vi "2100_Bridge_Read RFFE_w_Waveform_Publish Data.vi"(0 "Semiconductor Module Context":T2, 1 "Pins":string[](array[string])=["CLK", "SDA"], 2 "USID":T1=8 max=15, 3 "Reg Address":u8=6 format="%.0x", 5 "Error In":errorcluster, 6 "Read_Mode":enum16{"Reg_Read", "Bit_Read"}(ring), 7 "Bit_Location(LSB)":u8=7 max=7, 8 "Publish_Data?":bool, 9 "#ofBits":u8=1 min=1 max=8, 10 "Published Data Id":string) -> (14 "Converted Data":T3 {"Register" max=31 format="%.0x"; "Slave Address" max=15 format="%.0x"}, 15 "Reg Value":u8 format="%.0b", 19 "Error Out":errorcluster)   [LabVIEW 2013]
uses:
  <vilib>/NI_TestStand_SemiconductorModule/NI_TestStand_Semiconductor_Module.lvlibp/PinMap/General/SemiconductorModuleContext.ctl
  Controls/USID.ctl
  Controls/Reg_Address_Data.ctl
  <vilib>/NI_TestStand_SemiconductorModule/NI_TestStand_Semiconductor_Module.lvlibp/PinMap/General/Publish/PublishDataDoubleFunctionalTest.vi
  <vilib>/NI_TestStand_SemiconductorModule/NI_TestStand_Semiconductor_Module.lvlibp
panel:
  # "Specific Bit Readback"
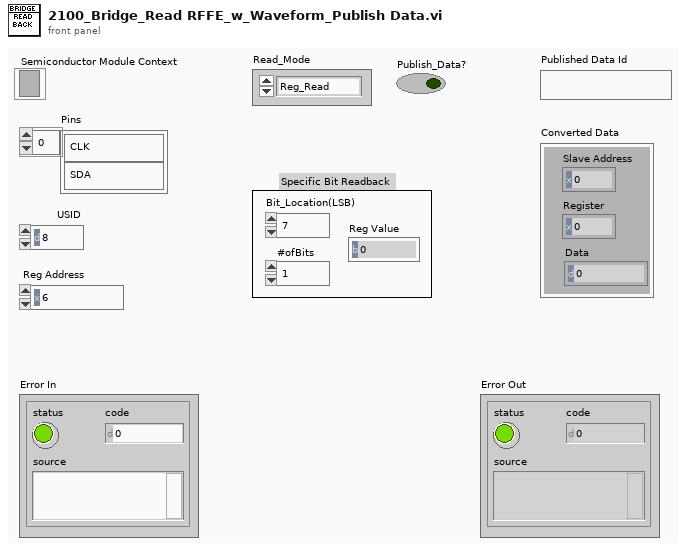
[diagram p1: front panel]
types:
  T1 = typedef "USID.ctl" = u8
  T2 = typedef "NI_TestStand_Semiconductor_Module.lvlibp/SemiconductorModuleContext.ctl" = refnum<k7>
  T3 = cluster{"Slave Address":u8, "Register":u8, "Data":u8}
  T4 = typedef "Reg_Address_Data.ctl" = cluster{"Address":u8, "Data":u8}
  T5 = cluster{"First Reg Address":u8, "Num of Reg to Read":u8}
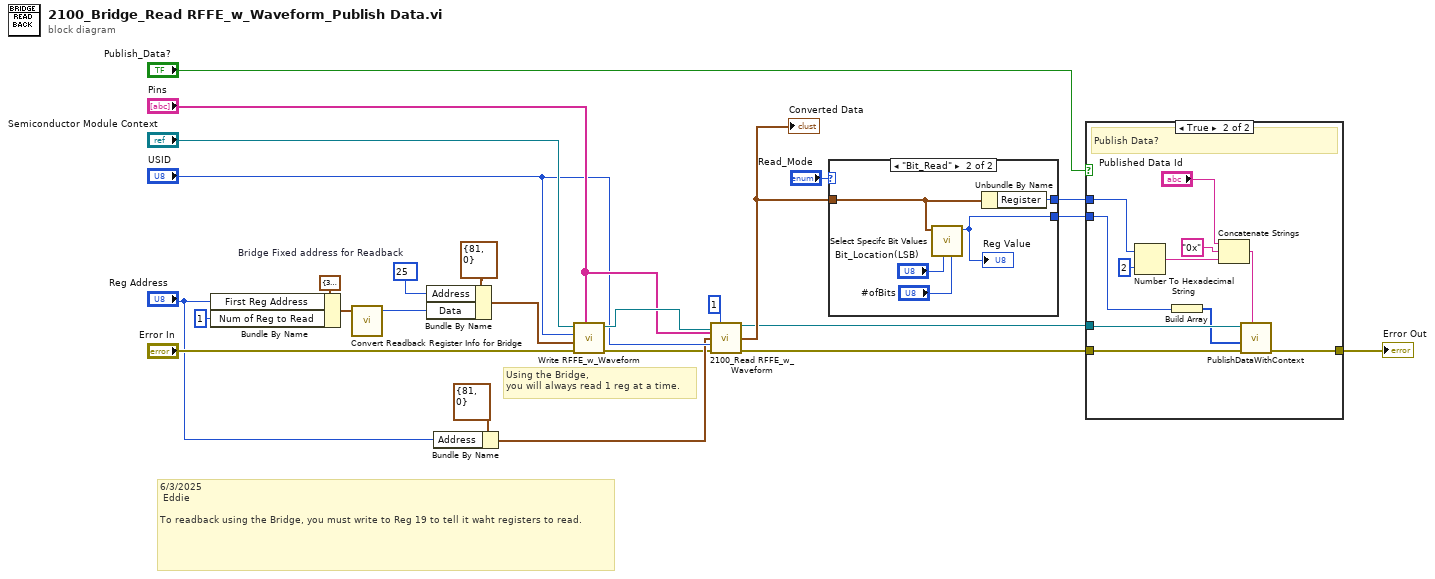
[diagram p0: block diagram]
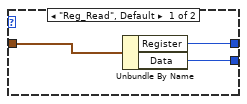
[diagram p2: hidden frame]
diagram:
  w23 = u8 25  # Bridge Fixed address for Readback
  # "Using the Bridge, \nyou will always read 1 reg at a time."
  # "6/3/2025\n Eddie\n\nTo readback using the Bridge, you must write to Reg 19 to tell it waht registers to read."
  n1 = Bundle By Name(cluster=T5 {"First Reg Address"=31, "Num of Reg to Read"=31} ("Reg_Address_to_Read"), "First Reg Address"="Reg Address", "Num of Reg to Read"=u8 1) -> (w14:T5)
  n2 = call "Convert Readback Register Info for Bridge.vi"("Reg_Address_to_Read"=w14) -> ("number"=w24:u32)  [unwired: 4 in]
  n3 = Bundle By Name(cluster=T4 {"Address"=81, "Data"=0} ("Reg_Address_Data"), "Address"=w23, "Data"=w24) -> (w21:T4)
  n4 = Bundle By Name(cluster=T4 {"Address"=81, "Data"=0} ("Reg_Address_Data"), "Address"="Reg Address") -> (w10:T4)
  n5 = call "Write RFFE_w_Waveform.vi"("Pins"="Pins", "error in (no error)"="Error In", "Reg_Address_Data"=w21, "USID"="USID", "Semiconductor Module Context"="Semiconductor Module Context") -> ("error out"=w9:errorcluster, "Semiconductor Module Context Out"=w19:T2)  [unwired: 5 in]
  n6 = call "2100_Read RFFE_w_Waveform.vi"("Semiconductor Module Context"=w19, "Num_Reg_to_Read"=u8 1, "Pins"="Pins", "Reg_Address_Data"=w10, "USID"="USID", "Error In"=w9) -> ("Semiconductor Module Context Out"=w1:T2, "Converted Data"=w4:T3, "Error Out"=w8:errorcluster)  [unwired: 7 in]
  "Converted Data" <- w4
  n7 = case shown="\"Bit_Read\"" "Read_Mode" {
    tunnel: w4 -> [w28 w31]
    tunnel: [w27 w30] -> w3
    tunnel: [w26 w29] -> w2
    frame "Reg_Read", Default {
      n8 = Unbundle By Name(w28) -> ("Register"=w27:u8, "Data"=w26:u8)
    }
    frame "Bit_Read" {
      n9 = call "Select Specifc Bit Values.vi"("#ofBits"="#ofBits", "Bit_Location(LSB)"="Bit_Location(LSB)", "Converted Data"=w31) -> ("Bits"=w29:u8)  [unwired: 8 in]
      "Reg Value" <- w29
      n10 = Unbundle By Name(w31) -> ("Register"=w30:u8)
    }
  }
  n11 = case shown="True" "Publish_Data?" {
    tunnel: [w34 w45] -> w6
    tunnel: w8 -> [w34 w44]
    tunnel: w2 -> [_ w42]
    tunnel: w3 -> [_ w41]
    tunnel: w1 -> [_ w39]
    frame False {
    }
    frame True {
      # "Publish Data?"
      n12 = Number To Hexadecimal String(1:i16 2 ("width (-)"), 2:w41) -> (0:w40:string)
      n13 = Build Array(w42) -> (w36:u8[])
      n14 = Concatenate Strings("Published Data Id", "0x" ("string"), w40) -> (w37:string)
      n15 = call-poly <vilib>:"PublishDataWithContext.vi"("Published Data Id"=w37, "error in (no error)"=w44, "Data In"=w36, "Semiconductor Module Context"=w39) -> ("error out"=w45:errorcluster)  [unwired: 6 in, 1 out]
    }
  }
  "Error Out" <- w6
